vi "Apply_h.vi"(4 "Noise Var":dbl, 6 "Input State":T1) -> (0 "y_r":dbl, 1 "y_c":dbl, 2 "m":dbl, 3 "h(x)":dbl[](array[numeric]))   [LabVIEW 2019]
uses:
  <vilib>/Analysis/NI_AALBase.lvlib
panel:
  out "Array 4":dbl[](array[numeric])
  out "Array 3":dbl[](array[numeric])
  out "Array 2":dbl[](array[numeric])
  out "Array":dbl[](array[numeric])
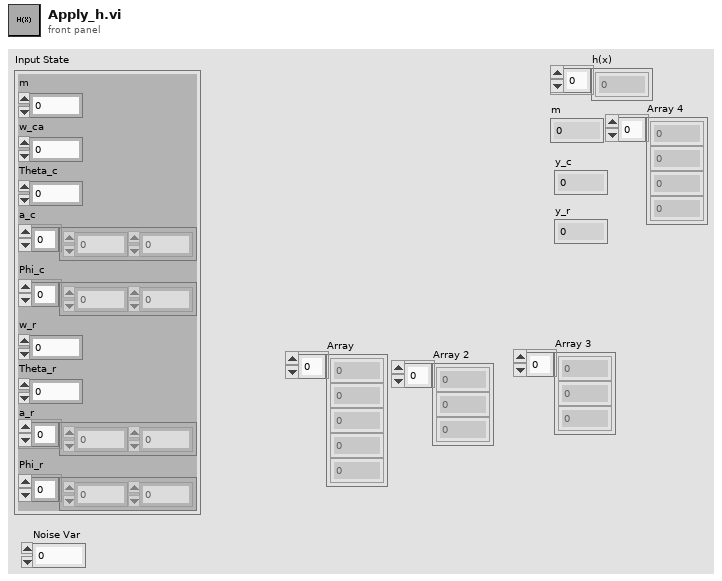
[diagram p1: front panel]
types:
  T1 = cluster{"m":dbl, "w_ca":dbl, "Theta_c":dbl, "a_c":dbl[], "Phi_c":dbl[], "w_r":dbl, "Theta_r":dbl, "a_r":dbl[], "Phi_r":dbl[]}
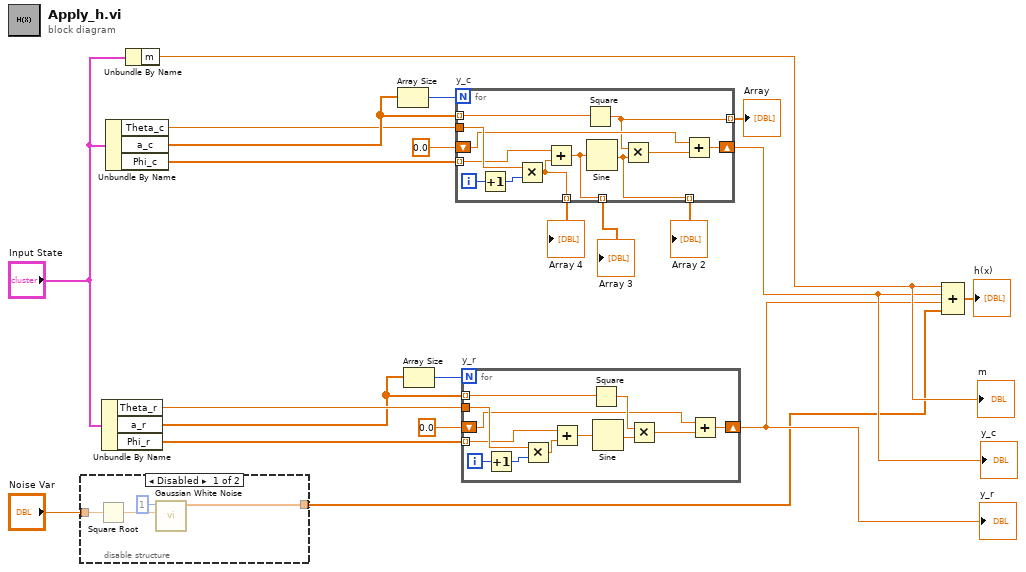
[diagram p0: block diagram]
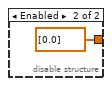
[diagram p2: hidden frame]
diagram:
  n1 = disable-structure shown="Disabled" {
    disable-tunnel: "Noise Var" -> [w25 _]
    disable-tunnel: [w22 dbl[] [0.0] ("Gaussian noise pattern")] -> w5
    frame Disabled {
      n2 = Square Root(x=w25) -> (sqrt(x)=w24:dbl)
      n3 = call <vilib>:"Gaussian White Noise.vi"("standard deviation"=w24, "samples"=1) -> ("Gaussian noise pattern"=w22:dbl[])  [unwired: 8 in, 1 out]
    }
    frame Enabled {
    }
  }
  n4 = Unbundle By Name("Input State") -> ("Theta_r"=w13:dbl, "a_r"=w12:dbl[], "Phi_r"=w11:dbl[])
  n5 = Unbundle By Name("Input State") -> ("Theta_c"=w18:dbl, "a_c"=w19:dbl[], "Phi_c"=w17:dbl[])
  n6 = Unbundle By Name("Input State") -> ("m"=w9:dbl)
  "m" <- w9
  n7 = Array Size(array=w19) -> (size(s)=w21:i32)
  n8 = Array Size(array=w12) -> (size(s)=w15:i32)
  n9 = for "y_c" {
    N: w21 -> [_]
    tunnel: w19 -> [w35] mode=indexing
    tunnel: w18 -> [w37]
    tunnel: w17 -> [w28] mode=indexing
    shift-right: [w36] -> w8
    shift-left: 0.0 -> [w34]
    tunnel: [w31] -> w4 mode=indexing
    tunnel: [w30] -> w3 mode=indexing
    tunnel: [w29] -> w2 mode=indexing
    tunnel: [w27] -> w1 mode=indexing
    i -> [w38]
    n10 = Increment(x=w38) -> (x+1=w33:i32)
    n11 = Multiply(x=w37, y=w33) -> (x*y=w27:dbl)
    n12 = Add(x=w28, y=w27) -> (x+y=w29:dbl)
    n13 = Square(x=w35) -> (x^2=w31:dbl)
    n14 = Sine(x=w29) -> (sin(x)=w30:dbl)
    n15 = Multiply(x=w31, y=w30) -> (x*y=w32:dbl)
    n16 = Add(x=w34, y=w32) -> (x+y=w36:dbl)
  }
  "y_c" <- w8
  "Array" <- w4
  "Array 2" <- w3
  "Array 3" <- w2
  "Array 4" <- w1
  n17 = for "y_r" {
    N: w15 -> [_]
    tunnel: w12 -> [w43] mode=indexing
    tunnel: w13 -> [w49]
    tunnel: w11 -> [w48] mode=indexing
    shift-right: [w45] -> w7
    shift-left: 0.0 -> [w42]
    i -> [w50]
    n18 = Increment(x=w50) -> (x+1=w40:i32)
    n19 = Multiply(x=w49, y=w40) -> (x*y=w47:dbl)
    n20 = Add(x=w48, y=w47) -> (x+y=w44:dbl)
    n21 = Square(x=w43) -> (x^2=w46:dbl)
    n22 = Sine(x=w44) -> (sin(x)=w41:dbl)
    n23 = Multiply(x=w46, y=w41) -> (x*y=w39:dbl)
    n24 = Add(x=w42, y=w39) -> (x+y=w45:dbl)
  }
  "y_r" <- w7
  n25 = Compound Arithmetic op=ADD(w9, w8, w7, w5) -> (→"h(x)":dbl[])
